vi "624 Fast Talon Set Voltage Ramp.vi"() -> ()   [LabVIEW 2015]
uses:
  <vilib>/Rock Robotics/WPI/MotorControl/WPI_MotorControlDeviceRef.ctl
  <vilib>/Rock Robotics/WPI/MotorControl/WPI_MotorControlType.ctl
  <vilib>/Rock Robotics/SystemInterfaces/DIO/FPGA_DIOPWMChannel.ctl
  <vilib>/Rock Robotics/WPI/PWM/WPI_PWMDeadband.ctl
  <vilib>/Rock Robotics/WPI/CAN/Jaguar/SubVIs/WPI_CANJaguar_ControlMode.ctl
  <vilib>/Rock Robotics/WPI/CAN/TalonSRX/WPI_CANTalonSRX_APIControlMode.ctl
  <vilib>/Rock Robotics/WPI/CAN/TalonSRX/WPI_CANTalonSRX_GlobalOps.ctl
  Common Code/Change Detect Double.vi
panel:
  in  "Throttle Ramp Rate (percent/s)":dbl
  out "error out":errorcluster
  in  "error in (no error)":errorcluster
  in  "CAN Talon SRX Ref":T1={"DeviceStatus"={"status"=FALSE, "code"=0, "source"=""}, "Type"=enum."PWM", "PWM"={"PWM Channel"=enum."PWM 1", "DeadBand"={"Name"="", "maxPositivePwm"=0, "minPositivePwm"=0, "centerPwm"=0, "maxNegativePwm"=0, "minNegativePwm"=0, "angularRange"=0}}, "CAN"={"Device Number"=0, "Control Mode"=enum."Percent VBus", "Semaphore"=refnum, "Max Vout"=12.0, "TalonSRX Control Mode"=enum."Percent VBus"}, "Invert"=FALSE}
  out "CAN Talon SRX Ref 2":T1={"DeviceStatus"={"status"=FALSE, "code"=0, "source"=""}, "Type"=enum."PWM", "PWM"={"PWM Channel"=enum."PWM 1", "DeadBand"={"Name"="", "maxPositivePwm"=0, "minPositivePwm"=0, "centerPwm"=0, "maxNegativePwm"=0, "minNegativePwm"=0, "angularRange"=0}}, "CAN"={"Device Number"=0, "Control Mode"=enum."Percent VBus", "Semaphore"=refnum, "Max Vout"=12.0, "TalonSRX Control Mode"=enum."Percent VBus"}, "Invert"=FALSE}
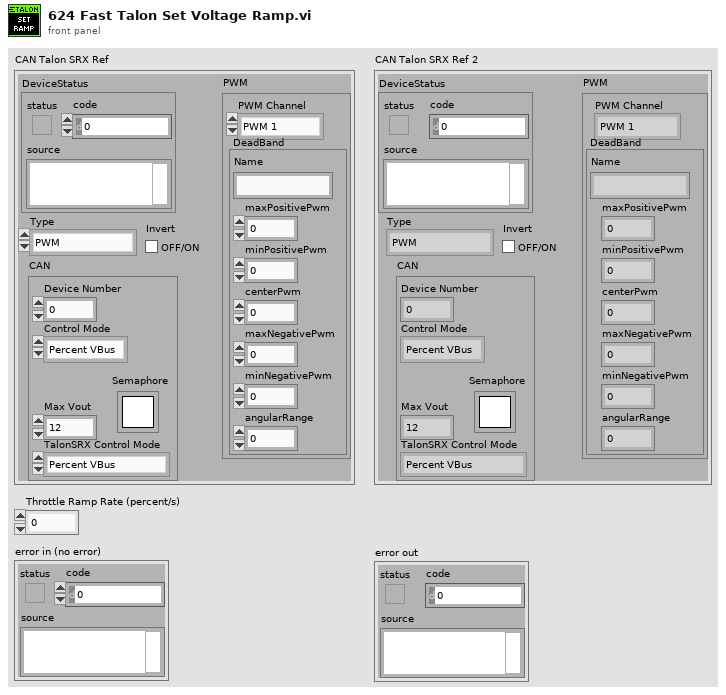
[diagram p1: front panel]
types:
  T1 = typedef "WPI_MotorControlDeviceRef.ctl" = cluster{"DeviceStatus":errorcluster, "Type":T2, "PWM":cluster{"PWM Channel":T3, "DeadBand":T4}, "CAN":cluster{"Device Number":u8, "Control Mode":T5, "Semaphore":T6, "Max Vout":dbl, "TalonSRX Control Mode":T7}, "Invert":bool}
  T2 = typedef "WPI_MotorControlType.ctl" = enum16{"PWM", "CAN", "CANTalonSRX"}
  T3 = typedef "FPGA_DIOPWMChannel.ctl" = enum8{"PWM 0", "PWM 1", "PWM 2", "PWM 3", "PWM 4", "PWM 5", "PWM 6", "PWM 7", "PWM 8", "PWM 9", "PWM MXP 0", "PWM MXP 1", "PWM MXP 2", "PWM MXP 3", "PWM MXP 4", "PWM MXP 5", "PWM MXP 6", "PWM MXP 7", "PWM MXP 8", "PWM MXP 9", "Invalid"}
  T4 = typedef "WPI_PWMDeadband.ctl" = cluster{"Name":string, "maxPositivePwm":i32, "minPositivePwm":i32, "centerPwm":i32, "maxNegativePwm":i32, "minNegativePwm":i32, "angularRange":u16}
  T5 = typedef "WPI_CANJaguar_ControlMode.ctl" = enum8{"Percent VBus", "Current", "Speed", "Position", "Voltage"}
  T6 = typedef "Semaphore RefNum" = refnum<k1>
  T7 = typedef "WPI_CANTalonSRX_APIControlMode.ctl" = enum8{"Percent VBus", "Speed", "Position", "Slave", "Unchanged / Invalid", "Voltage Compensation", "Current", "Motion Profile"}
  T8 = typedef "WPI_CANTalonSRX_GlobalOps.ctl" = enum16{"Read For Send", "Write After Receive General", "Write After Receive Feedback", "Write After Receive Encoder", "Write After Receive Ain", "Write Error", "Get All", "Set Output", "Set Mode", "Set Master ID", "Set Brake Mode", "Set Reverse Feedback Sensor", "Set Reverse Closed Loop Output", "Set Override Limits", "Set Forward Limit Enabled", "Set Reverse Limit Enabled", "Set Feedback Select", "Set Profile Select", "Set Throttle Ramp Rate", "Disable", "Set Enc Codes Per Rev", "Set Num Pot Turns", "Set Control Frame Rate", "Enable Legacy Control", "Write After Receive Pulse Width", "Set Enable Frame Rate", "Write After Receive Motion Profile", "Set Motion Profile Flow Control", "Set Motion Profile Control Frame Rate"}
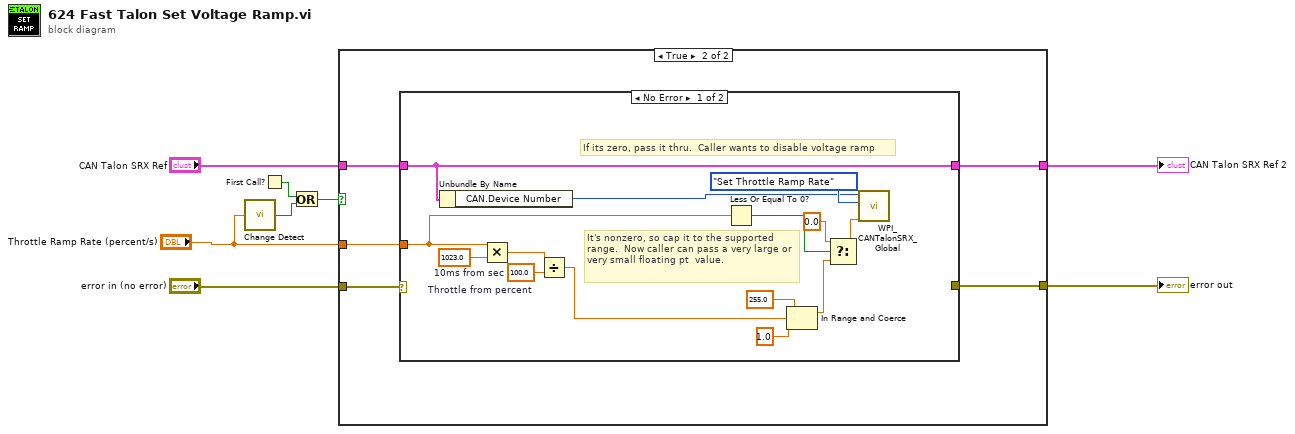
[diagram p0: block diagram]
diagram:
  n1 = call-poly "Change Detect.vi"("In"="Throttle Ramp Rate (percent/s)") -> ("Changed?"=w3:bool)
  n2 = First Call?() -> (First Call?: T/F=w2:bool)
  n3 = Or(x=w2, y=w3) -> (x .or. y?=w1:bool)
  n4 = case shown="True" w1 {
    tunnel: [w9 w15] -> w8
    tunnel: "error in (no error)" -> [w9 w14]
    tunnel: [w10 w13] -> w6
    tunnel: "CAN Talon SRX Ref" -> [w10 w12]
    tunnel: "Throttle Ramp Rate (percent/s)" -> [_ w11]
    frame False {
    }
    frame True {
      n5 = case shown="No Error" w14 {
        selector: w14 -> [_ w31]
        tunnel: [_ w31] -> w15
        tunnel: [w29 w30] -> w13
        tunnel: w12 -> [w29 w30]
        tunnel: w11 -> [w22 _]
        frame No Error {
          w26 = 100.0  # 10ms from sec
          w28 = 1023.0  # Throttle from percent
          # "It's nonzero, so cap it to the supported range.  Now caller can pass a very large or very small floating pt  value."
          # "If its zero, pass it thru.  Caller wants to disable voltage ramp"
          n6 = Unbundle By Name(w29) -> ("CAN.Device Number"=w17:u8)
          n7 = Multiply(x=w22, y=w28) -> (x*y=w27:dbl)
          n8 = Divide(x=w27, y=w26) -> (x/y=w20:dbl)
          n9 = Less Or Equal To 0?(x=w22) -> (x <= 0?=w24:bool)
          n10 = In Range and Coerce(upper limit=255.0, x=w20, lower limit=1.0) -> (coerced(x)=w19:dbl)  [unwired: 1 out]
          n11 = Select(t=0.0, s=w24, f=w19) -> (s? t:f=w16:dbl)
          n12 = call <vilib>:"WPI_CANTalonSRX_Global.vi"("Set Number"=w16, "Operation"=WPI_CANTalonSRX_GlobalOps."Set Throttle Ramp Rate", "Device ID (0)"=w17) -> ()  [unwired: 6 in, 3 out]
        }
        frame Error {
        }
      }
    }
  }
  "CAN Talon SRX Ref 2" <- w6
  "error out" <- w8
